vi "StartCamera.vi"(0 "Parameteres":T1, 1 "Error in":errorcluster) -> (2 "camera":refnum<class "CameraBase.lvclass">, 3 "params":variant, 4 "error out":errorcluster)   [LabVIEW 2012]
uses:
  <userlib>/bias2/classes/CameraBase/CameraBase.lvclass
  <userlib>/bias2/subvis/ui/CameraParameters.ctl
  <userlib>/_OpenG.lib/error/error.llb/Filter Error Codes (Array)__ogtk.vi
  <vilib>/addons/h5labview/H5File.lvlib
  <vilib>/addons/h5labview/H5Attrib.lvlib
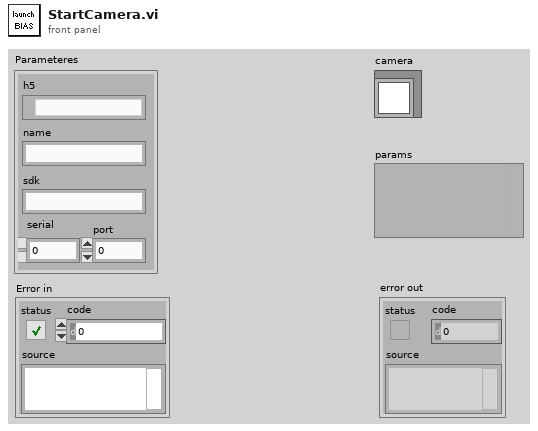
[diagram p1: front panel]
types:
  T1 = typedef "CameraParameters.ctl" = cluster{"name":string, "sdk":string, "serial":u64, "port":u16, "h5":path}
  T2 = typedef "CameraInfo.ctl" = cluster{"name":string, "serial":u64, "interface":string, "make":string, "model":string, "pixel_w":dbl, "pixel_h":dbl}
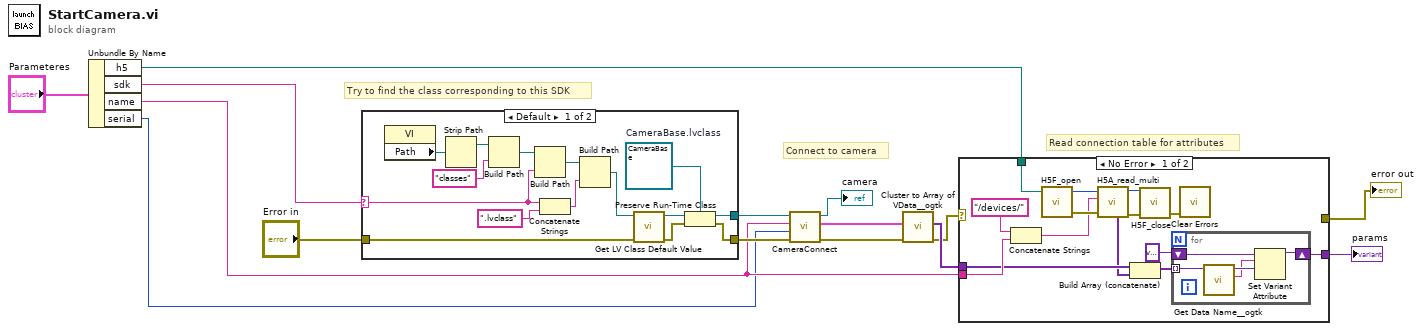
[diagram p0: block diagram]
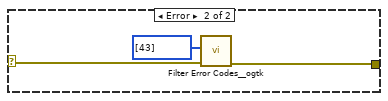
[diagram p3: hidden frame]
diagram:
  # "Connect to camera"
  # "Try to find the class corresponding to this SDK"
  # "Read connection table for attributes"
  n1 = Unbundle By Name("Parameteres") -> ("h5"=w4:path, "sdk"=w3:string, "name"=w2:string, "serial"=w1:u64)
  n2 = case shown="Default" w3 {
    selector: w3 -> [w24 _]
    tunnel: [w20 _] -> w13
    tunnel: "Error in" -> [w18 w31]
    tunnel: [w17 w31] -> w12
    frame Default {
      w16 = refnum<class "CameraBase.lvclass"> refnum  # CameraBase.lvclass
      n3 = property on="Property Node" class="VI"() -> ("Path"=w30:path)  [unwired: 2 in, 2 out]
      n4 = Strip Path(path=w30) -> (stripped path=w29:path)  [unwired: 1 out]
      n5 = Build Path(base path=w29, name or relative path="classes") -> (appended path=w27:path)
      n6 = Build Path(base path=w27, name or relative path=w24) -> (appended path=w26:path)
      n7 = Concatenate Strings(w24, ".lvclass" ("string")) -> (w23:string)
      n8 = Build Path(base path=w26, name or relative path=w23) -> (appended path=w25:path)
      n9 = call <vilib>:"Get LV Class Default Value.vi"("error in (no error)"=w18, "class path"=w25) -> ("error out"=w19:errorcluster, "object"=w21:refnum<class>)  [unwired: 8 in]
      n10 = Preserve Run-Time Class(object in=w21, error in=w19, 2:w16) -> (object out=w20:refnum<class "CameraBase.lvclass">, error out=w17:errorcluster)
    }
    frame "" {
      # "Cancelled OR offline"
    }
  }
  n11 = call-dynamic "CameraConnect.vi"("error in (no error)"=w12, "serial"=w1, "name"=w2, "CameraBase in"=w13) -> ("error out"=w7:errorcluster, "CameraInfo"=w10:T2, "CameraBase out"=→"camera":refnum<class "CameraBase.lvclass">)  [unwired: 5 in]
  n12 = call <userlib>:"Cluster to Array of VData__ogtk.vi"("error in (no error)"=w7, "Cluster"=w10) -> ("error out"=w8:errorcluster, "Array of VData"=w9:variant[])  [unwired: 8 in]
  n13 = case shown="No Error" w8 {
    selector: w8 -> [_ w53]
    tunnel: w4 -> [w45 _]
    tunnel: w2 -> [w37 _]
    tunnel: [_ w52] -> w6
    tunnel: [w36 _] -> w15
    tunnel: w9 -> [w35 _]
    frame No Error {
      n14 = Concatenate Strings("/devices/", w37) -> (w39:string)
      n15 = call <vilib>:"H5F_open.vi"("path"=w45) -> ("error out"=w41:errorcluster, "ref"=w43:i32)  [unwired: 3 in]
      n16 = call <vilib>:"H5A_read_multi.vi"("error in (no error)"=w41, "obj_name"=w39, "ref"=w43) -> ("error out"=w40:errorcluster, "ref out"=w42:i32, "attribs"=w34:variant[])  [unwired: 4 in]
      n17 = Build Array (concatenate)(w35, w34) -> (w33:variant[])
      n18 = call <vilib>:"H5F_close.vi"("error in (no error)"=w40, "ref"=w42) -> ("error out"=w38:errorcluster)  [unwired: 3 in]
      n19 = for {
        tunnel: w33 -> [w48] mode=indexing
        shift-right: [w47] -> w36
        shift-left: variant ("1D Array of Variants") -> [w46]
        n20 = call <userlib>:"Get Data Name__ogtk.vi"("Data"=w48) -> ("Data Name"=w49:string, "Data dup"=w50:variant)  [unwired: 8 in, 1 out]
        n21 = Set Variant Attribute(Variant=w46, name=w49, value=w50) -> (Variant out=w47:variant)  [unwired: 1 in, 2 out]
      }
      n22 = call <vilib>:"Clear Errors.vi"("error in (no error)"=w38) -> ()  [unwired: 6 in, 1 out]
    }
    frame Error {
      n23 = call-poly <userlib>:"Filter Error Codes__ogtk.vi"("Error In"=w53, "Error Codes to Filter"=i32[] [43]) -> ("Error Out"=w52:errorcluster)  [unwired: 7 in, 2 out]
    }
  }
  "params" <- w15
  "error out" <- w6
